vi "Highlight Top SubVI.vi"(8 "error in (no error)":errorcluster, 11 "Data in":T1={"PeekVI Reference"=refnum, "SubPanel"=refnum, "Peek Stack Tree Ref"=refnum, "Open Button Ref"=refnum, "Top VI"=refnum, "Active VI"=refnum, "Stack"=[], "Last FP State"=enum."Standard"}) -> (0 "error out":errorcluster, 3 "Data out":T1={"PeekVI Reference"=refnum, "SubPanel"=refnum, "Peek Stack Tree Ref"=refnum, "Open Button Ref"=refnum, "Top VI"=refnum, "Active VI"=refnum, "Stack"=[], "Last FP State"=enum."Standard"})   [LabVIEW 2020, in "Peek Window.lvlib"]
uses:
  Peek Window.lvlib
  MHL Data Cluster.ctl
  VI Types/Standard VI Type/Standard VI Type.lvclass
  VI Types/Standard VI Type/Standard VI Type.lvclass/Standard VI Type.ctl
  Symbols Enum.ctl
  VI Types/Standard VI Type/Read VI Refnum.vi
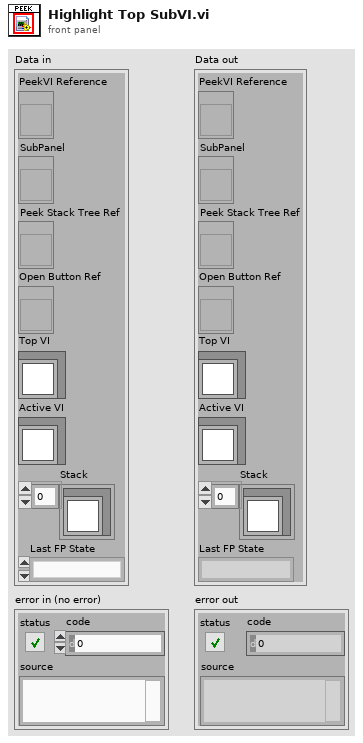
[diagram p1: front panel]
types:
  T1 = typedef "Peek Window.lvlib/MHL Data Cluster.ctl" = cluster{"PeekVI Reference":refnum<vi>, "SubPanel":refnum<vi>, "Peek Stack Tree Ref":refnum<vi>, "Open Button Ref":refnum<vi>, "Top VI":refnum<class "Standard VI Type.lvclass">, "Active VI":refnum<class "Standard VI Type.lvclass">, "Stack":refnum<class "Standard VI Type.lvclass">[], "Last FP State":enum32{"Invalid", "Standard", "Closed", "Hidden", "Minimized", "Maximized"}}
  T2 = typedef "Peek Window.lvlib/Symbols Enum.ctl" = enum16{"<Blank>", "Implementation Mark", "Standard VI", "Dynamic Dispatch VI", "Malleable VI", "Polymorphic VI", "Missing VI", "Express VI"}
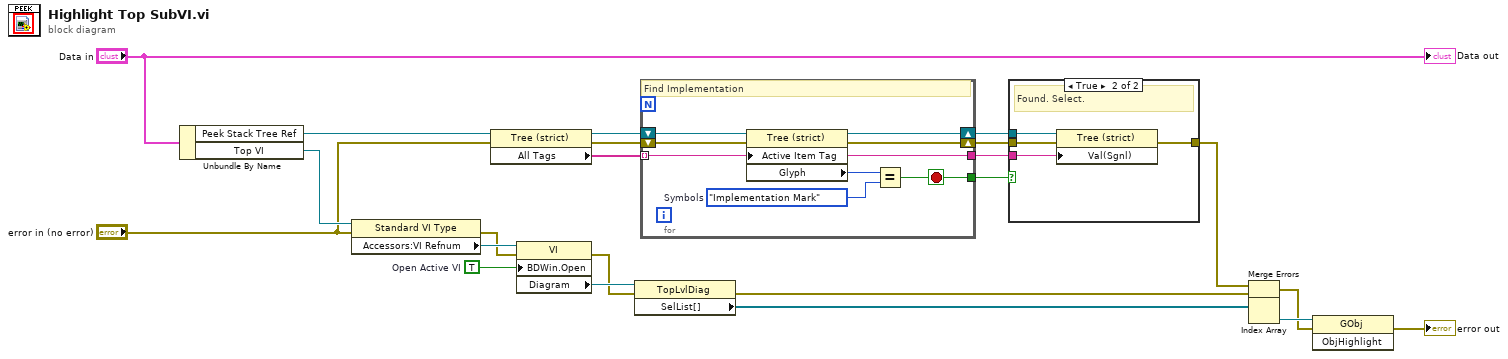
[diagram p0: block diagram]
diagram:
  w21 = TRUE  # Open Active VI
  n1 = Unbundle By Name("Data in") -> ("Peek Stack Tree Ref"=w11:refnum<vi>, "Top VI"=w15:refnum<class "Standard VI Type.lvclass">)
  n2 = property class="Standard VI Type"(reference=w15, error in="error in (no error)") -> (error out=w13:errorcluster, "Accessors:VI Refnum"=w14:refnum<vi>)  [unwired: 1 out]
  n3 = property class="Tree (strict)"(reference=w11, error in="error in (no error)") -> (reference out=w8:refnum<vi>, error out=w9:errorcluster, "All Tags"=w2:string[])
  n4 = property class="VI"(reference=w14, error in=w13, "BDWin.Open"=w21) -> (error out=w17:errorcluster, "Diagram"=w18:refnum<vi>)  [unwired: 1 out]
  n5 = property class="TopLvlDiag"(reference=w18, error in=w17) -> (error out=w16:errorcluster, "SelList[]"=w20:refnum<vi>[])  [unwired: 1 out]
  n6 = for {
    tunnel: [w24] -> w5
    tunnel: w2 -> [w23] mode=indexing
    shift-right: [w27] -> w6
    shift-left: w9 -> [w30]
    shift-right: [w28] -> w7
    shift-left: w8 -> [w29]
    tunnel: [w23] -> w1
    stop <- w24 stop-if-true
    w25 = Symbols_Enum."Implementation Mark"  # Symbols
    # "Find Implementation"
    n7 = property class="Tree (strict)"(reference=w29, error in=w30, "Active Item Tag"=w23) -> (reference out=w28:refnum<vi>, error out=w27:errorcluster, "Glyph"=w26:i32)
    n8 = Equal?(x=w26, y=w25) -> (x = y?=w24:bool)
  }
  n9 = case shown="True" w5 {
    tunnel: w7 -> [_ w35]
    tunnel: w6 -> [w31 w34]
    tunnel: w1 -> [_ w33]
    tunnel: [w31 w32] -> w3
    frame False {
      # "None. Do Nothing."
    }
    frame True {
      # "Found. Select."
      n10 = property class="Tree (strict)"(reference=w35, error in=w34, "Val(Sgnl)"=w33) -> (error out=w32:errorcluster)  [unwired: 1 out]
    }
  }
  n11 = Merge Errors(w3, w16) -> (w4:errorcluster)
  n12 = Index Array(array=w20) -> (element=w19:refnum<vi>)  [unwired: 1 in]
  n13 = invoke class="GObj" method="ObjHighlight"(reference=w19, error in=w4) -> (error out=→"error out":errorcluster)  [unwired: 1 in, 2 out]
  "Data out" <- "Data in"
